vi "CalcIntTime.vi"(9 "Int Time":i32[](array[numeric]), 11 "Array":dbl[](array[numeric])) -> (1 "IntegrationTime":dbl, 2 "Saturated? 2":bool, 3 "Saturated?":bool)   [LabVIEW 2012]
uses:
  <vilib>/gmath/NI_Gmath.lvlib
panel:
  out "appended array":dbl[](array[numeric])
  out "xi used":dbl[](array[numeric]) format="%_6g"
  out "yi":dbl[](array[numeric]) format="%_6g"
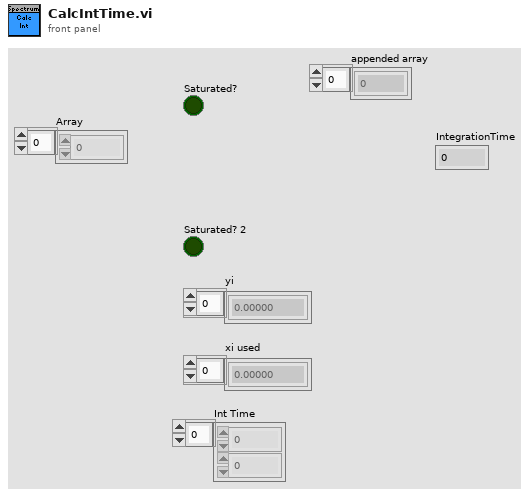
[diagram p1: front panel]
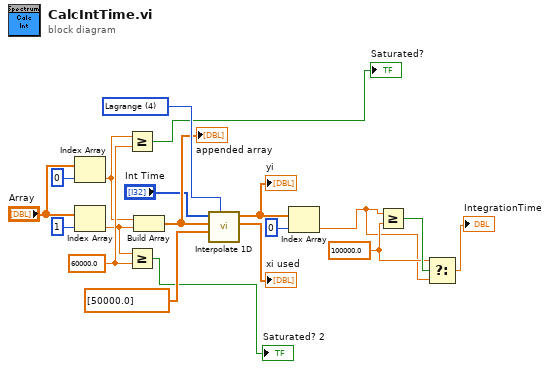
[diagram p0: block diagram]
diagram:
  w3 = 100000.0 ("y")
  w19 = 4 items=["nearest", "linear", "spline", "cubic Hermite", "Lagrange"] ("method")
  w10 = 60000.0 ("y")
  n1 = Index Array(array="Array", index=0) -> (element=w6:dbl)
  n2 = Index Array(array="Array", index=1) -> (element=w5:dbl)
  n3 = Greater Or Equal?(x=w6, y=w10) -> (x >= y?=→"Saturated?":bool)
  n4 = Greater Or Equal?(x=w5, y=w10) -> (x >= y?=→"Saturated? 2":bool)
  n5 = Build Array(w6, w5) -> (w15:dbl[])
  "appended array" <- w15
  n6 = call <vilib>:"Interpolate 1D.vi"("method"=w19, "xi"=dbl[] [50000.0], "X"=w15, "Y"="Int Time") -> ("xi used"=→"xi used":dbl[], "yi"=w13:dbl[])  [unwired: 5 in, 1 out]
  "yi" <- w13
  n7 = Index Array(array=w13, index=0) -> (element=w2:dbl)
  n8 = Greater Or Equal?(x=w2, y=w3) -> (x >= y?=w4:bool)
  n9 = Select(t=w3, s=w4, f=w2) -> (s? t:f=→"IntegrationTime":dbl)
